vi "Download Album Image.vi"(8 "error in (no error)":errorcluster, 10 "Song":refnum<class "Song.lvclass">, 11 "AlbumImageActor in":refnum<class "AlbumImageActor.lvclass">) -> (0 "error out":errorcluster, 3 "AlbumImageActor out":refnum<class "AlbumImageActor.lvclass">)   [LabVIEW 2015, in "AlbumImageActor.lvlib" / "AlbumImageActor.lvclass"]
uses:
  AlbumImageActor.lvclass
  file/MusicElement/Song/Song.lvclass
  file/MusicElement/Song/Song.lvclass/Song.ctl
  AlbumImageActor.lvclass/AlbumImageActor.ctl
  <vilib>/httpClient/LabVIEWHTTPClient.lvlib
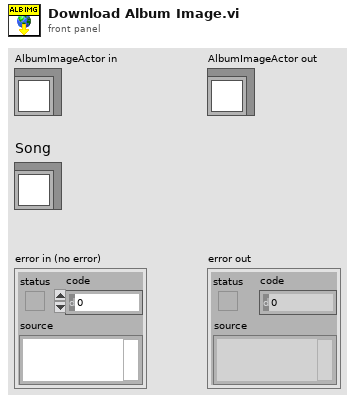
[diagram p1: front panel]
types:
  T1 = typedef "LabVIEWHTTPClient.lvlib/ClientHandle.ctl" = refnum<k1>
  T2 = typedef "imagedata.ctl" = cluster{"image type":i32, "image depth":i32, "image":u8[], "mask":u8[], "colors":u32[], "Rectangle":cluster{"left":i16, "top":i16, "right":i16, "bottom":i16}}
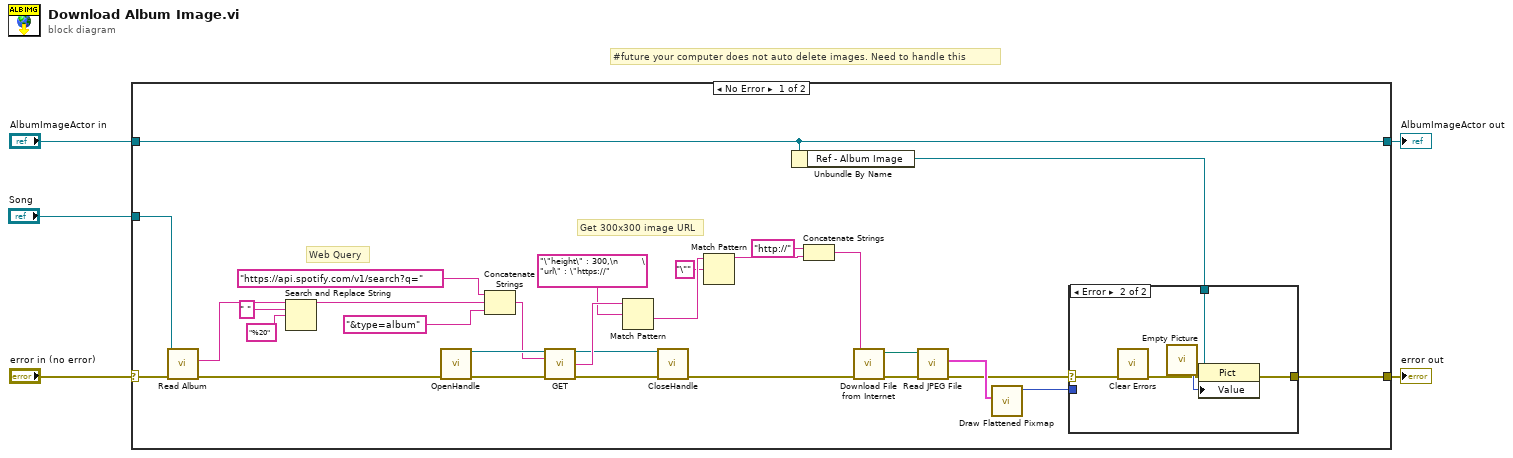
[diagram p0: block diagram]
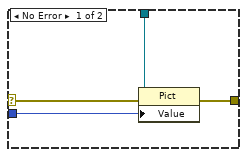
[diagram p2: hidden frame]
diagram:
  # "#future your computer does not auto delete images. Need to handle this"
  n1 = case shown="No Error" "error in (no error)" {
    selector: "error in (no error)" -> [w9 w46]
    tunnel: [w6 w46] -> w4
    tunnel: [w18 w45] -> w2
    tunnel: "AlbumImageActor in" -> [w18 w45]
    tunnel: "Song" -> [w20 _]
    frame No Error {
      # "Get 300x300 image URL"
      # "Web Query"
      n2 = call "Read Album.vi"("error in (no error)"=w9, "Song in"=w20) -> ("error out"=w10:errorcluster, "Album"=w19:string)  [unwired: 7 in, 1 out]
      n3 = Search and Replace String(input string=w19, search string=" ", replace string="%20" ("replace string (\"\")")) -> (result string=w32:string)  [unwired: 5 in, 3 out]
      n4 = call <vilib>:"OpenHandle.vi"("error in (no error)"=w10) -> ("client handle out"=w30:T1, "error out"=w11:errorcluster)  [unwired: 13 in]
      n5 = Concatenate Strings("https://api.spotify.com/v1/search?q=" ("url"), w32, "&type=album" ("url")) -> (w29:string)
      n6 = call <vilib>:"GET.vi"("client handle"=w30, "url"=w29, "error in (no error)"=w11) -> ("client handle out"=w22:T1, "body"=w28:string, "error out"=w12:errorcluster)  [unwired: 9 in, 1 out]
      n7 = Match Pattern(string=w28, regular expression="\"height\" : 300,\n        \"url\" : \"https://" ("url")) -> (after substring=w26:string)  [unwired: 1 in, 3 out]
      n8 = call <vilib>:"CloseHandle.vi"("client handle"=w22, "error in (no error)"=w12) -> ("error out"=w8:errorcluster)  [unwired: 13 in]
      n9 = Match Pattern(string=w26, regular expression="\"") -> (before substring=w24:string)  [unwired: 1 in, 3 out]
      n10 = Unbundle By Name(w18) -> ("Ref - Album Image"=w15:refnum<vi>)
      n11 = Concatenate Strings("http://" ("string"), w24) -> (w21:string)
      n12 = call "Download File from Internet.vi"("Error In"=w8, "URL to File"=w21) -> ("Error Out"=w13:errorcluster, "Downloaded File"=w16:path)  [unwired: 3 in, 1 out]
      n13 = call <vilib>:"Read JPEG File.vi"("error in (no error)"=w13, "path to JPEG file"=w16) -> ("error out"=w14:errorcluster, "image data"=w17:T2)  [unwired: 8 out]
      n14 = call <vilib>:"Draw Flattened Pixmap.vi"("image data"=w17) -> ("new picture"=w7:picture)  [unwired: 1 in, 7 out]
      n15 = case shown="Error" w14 {
        selector: w14 -> [w37 w41]
        tunnel: w15 -> [w39 w43]
        tunnel: w7 -> [w38 _]
        tunnel: [w36 w44] -> w6
        frame No Error {
          n16 = property class="Pict"(reference=w39, error in=w37, "Value"=w38) -> (error out=w36:errorcluster)  [unwired: 1 out]
        }
        frame Error {
          n17 = call <vilib>:"Clear Errors.vi"("error in (no error)"=w41) -> ("error out"=w40:errorcluster)  [unwired: 5 in, 1 out]
          n18 = call "Empty Picture"() -> ("empty picture"=w42:picture)
          n19 = property class="Pict"(reference=w43, error in=w40, "Value"=w42) -> (error out=w44:errorcluster)  [unwired: 1 out]
        }
      }
    }
    frame Error {
    }
  }
  "error out" <- w4
  "AlbumImageActor out" <- w2
